vi "Measure Bio Type2String.vi"(8 "error in (no error)":errorcluster caption="错误输入（无错误）", 11 "Measure_Bio_Type Input":T1[](array[typedef])) -> (0 "error out":errorcluster caption="错误输出", 3 "Measure Bio Type":string[][](array[string]))   [LabVIEW 2015, in "Utility VIs.lvlib"]
doc: "该模板用于创建子VI。"
uses:
  Utility VIs.lvlib
  Database Processing/Support/Table/Measure_Bio_Type.ctl
  Database Processing/Database Processing.lvlib
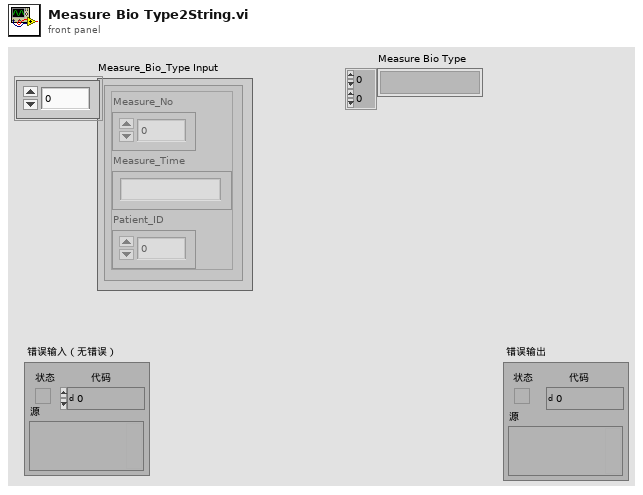
[diagram p1: front panel]
types:
  T1 = typedef "Database Processing.lvlib/Measure_Bio_Type.ctl" = cluster{"Measure_No":i64, "Measure_Time":string, "Patient_ID":i64}
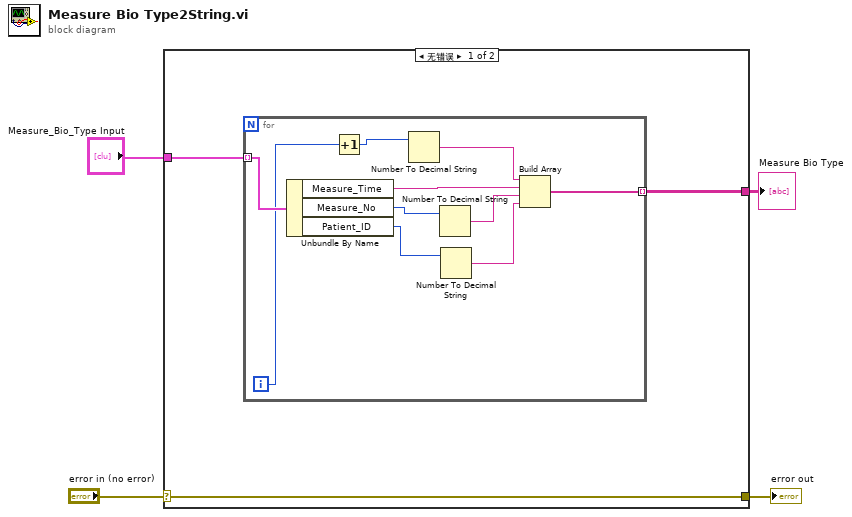
[diagram p0: block diagram]
diagram:
  n1 = case shown="无错误" "error in (no error)" {
    selector: "error in (no error)" -> [w6 w18]
    tunnel: [w6 w18] -> w3
    tunnel: "Measure_Bio_Type Input" -> [w7 _]
    tunnel: [w5 _] -> w2
    frame No Error {
      n2 = for {
        tunnel: w7 -> [w17] mode=indexing
        tunnel: [w14] -> w5 mode=indexing
        i -> [w8]
        n3 = Unbundle By Name(w17) -> ("Measure_Time"=w15:string, "Measure_No"=w13:i64, "Patient_ID"=w11:i64)
        n4 = Increment(x=w8) -> (x+1=w9:i32)
        n5 = Number To Decimal String(number=w9) -> (decimal integer string=w16:string)  [unwired: 1 in]
        n6 = Number To Decimal String(number=w13) -> (decimal integer string=w12:string)  [unwired: 1 in]
        n7 = Number To Decimal String(number=w11) -> (decimal integer string=w10:string)  [unwired: 1 in]
        n8 = Build Array(w16, w15, w12, w10) -> (w14:string[])
      }
    }
    frame Error {
    }
  }
  "error out" <- w3
  "Measure Bio Type" <- w2
